vi "_cameras_right_hand_camera_image(Jed)Subscriber_Server.vi"() -> ()   [LabVIEW 2012]
uses:
  <userlib>/rosforlv/ROS/Code/SubVIs/_ROSControl.ctl
  <userlib>/rosforlv/ROS/Code/SubVIs/_ROSDirection.ctl
  <userlib>/rosforlv/ROS/Code/Console/Servers/ServerSubs/ROSLog.ctl
  <userlib>/rosforlv/ROS/Code/Console/Servers/ServerSubs/MyState.ctl
  <userlib>/rosforlv/ROS/Code/Console/Servers/ServerSubs/requestTopic.ctl
panel:
  out "Log of port":string
  out "Queue log":string
  out "Last Reply":string
  out "Registered topics":T1[](array[typedef])
  out "Registering":bool
  out "MyState":T3
  out "(Un)Reg Text":string
  out "Setup":string
  out "Cmd Log":T4[](array[typedef])
  out "Connections Error log":string
  out "Connections":T5(array[cluster])
  out "Error log":string
  in  "stop":bool
  in  "ROS":T1={"topic port"=1236, "Node"="/labview", "topic"="/robot/head/command_head_nod", "type"="std_msgs/Bool", "node port"=7000, "error "={"status"=FALSE, "code"=0, "source"=""}, "Direction"=enum."Publisher", "APIs"=[], "Update (ms)"=1, "write queue"=1}
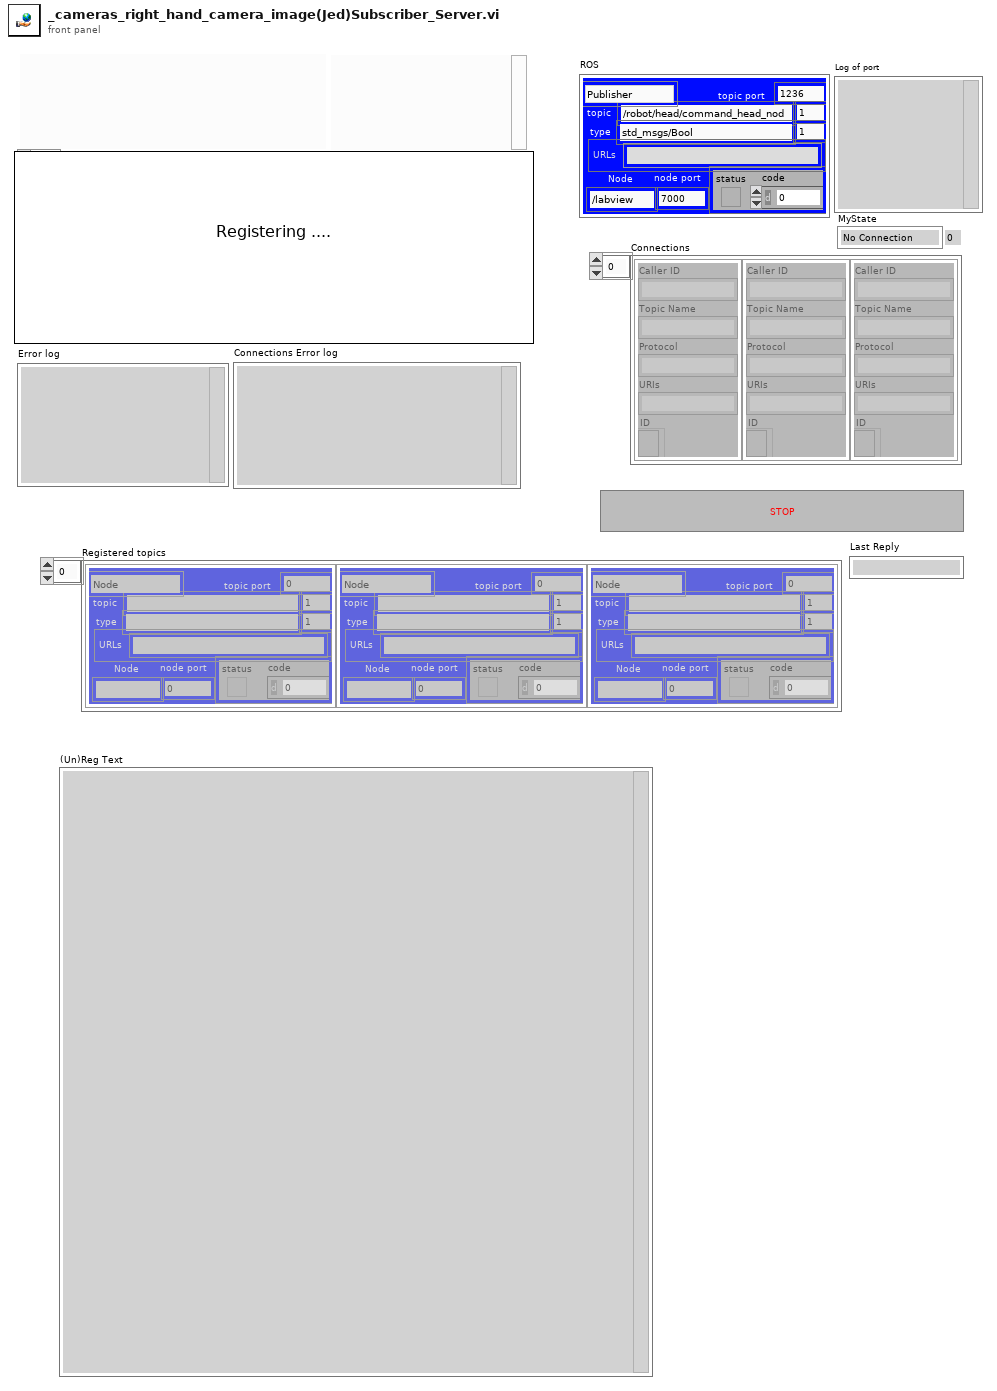
[diagram p1: front panel]
types:
  T1 = typedef "_ROSControl.ctl" = cluster{"topic port":u16, "Node":string, "topic":string, "type":string, "node port":u32, "error ":errorcluster, "Direction":T2, "APIs":string[], "Update (ms)":u16, "write queue":u16}
  T2 = typedef "_ROSDirection.ctl" = enum16{"Node", "Publisher", "Subscriber", "Service Client"}
  T3 = typedef "MyState.ctl" = enum16{"No Connection", "Registered", "Connected", "Close"}
  T4 = typedef "ROSLog.ctl" = cluster{"Sent":string, "Reply":string, "MethodName":string, "success":bool, "Dir1":string, "Dir2":string, "Time Stamp":string}
  T5 = cluster{"Caller ID":string, "Topic Name":string, "Protocol":string, "URIs":string, "ID":refnum<k5>}[]
  T6 = typedef "requestTopic.ctl" = cluster{"New Subscriber":cluster{"Caller ID":string, "Topic Name":string, "Protocol":string, "URIs":string, "ID":refnum<k5>}, "ROS of Server":T1, "new port":u16}
  T7 = cluster{"Code":i32, "Status Message":string, "APIs":string[]}
  T8 = cluster{"Caller ID":string, "Topic Name":string, "Protocol":string, "URIs":string, "ID":refnum<k5>}
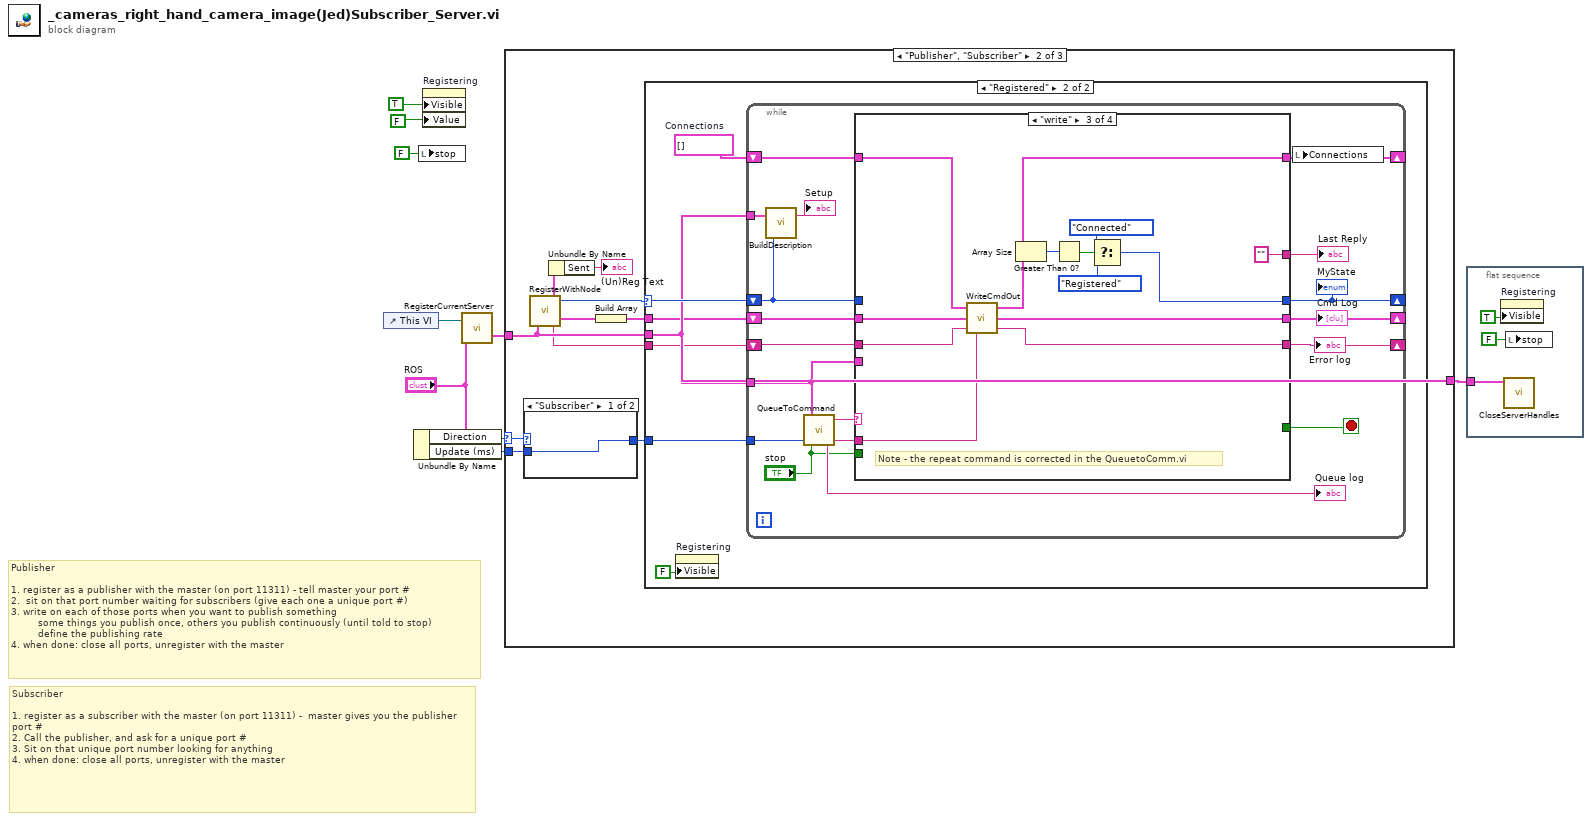
[diagram p0: block diagram]
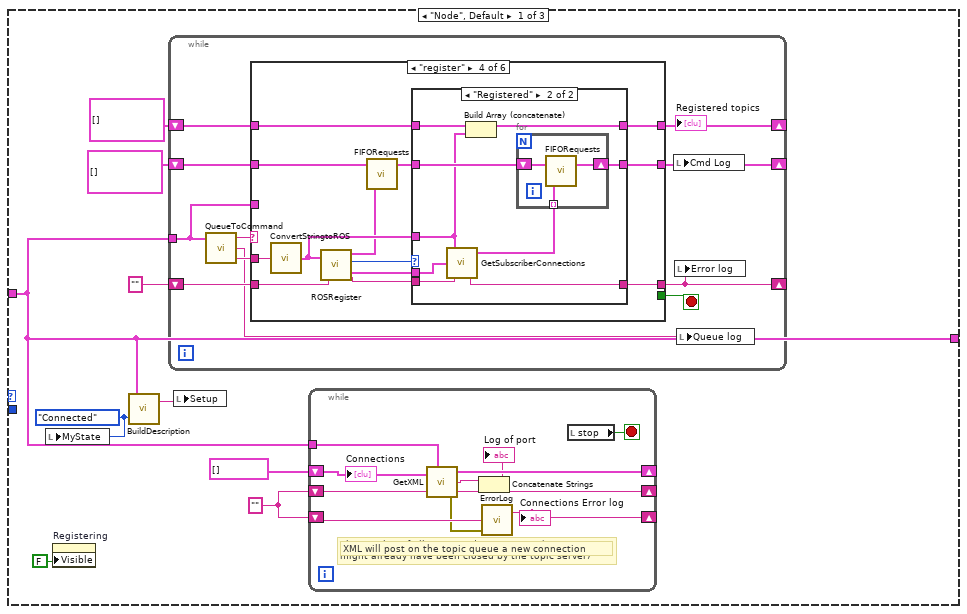
[diagram p2: hidden frame]
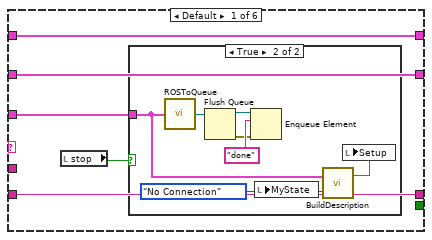
[diagram p3: hidden frame]
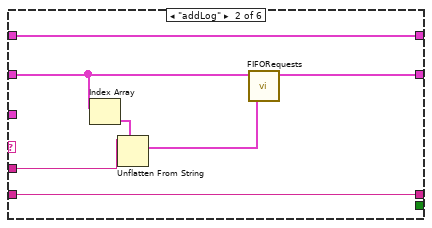
[diagram p5: hidden frame]
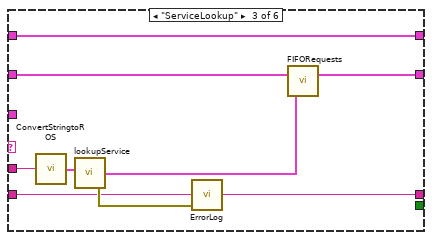
[diagram p6: hidden frame]
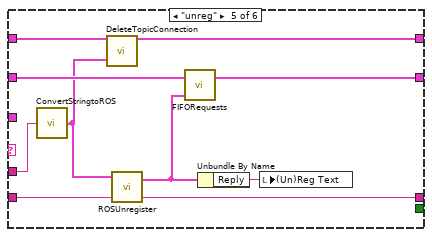
[diagram p8: hidden frame]
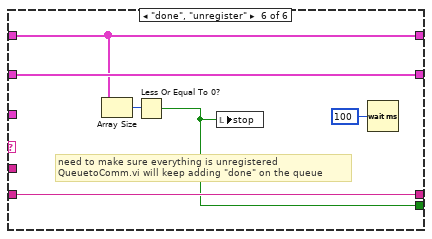
[diagram p9: hidden frame]
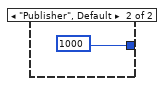
[diagram p10: hidden frame]
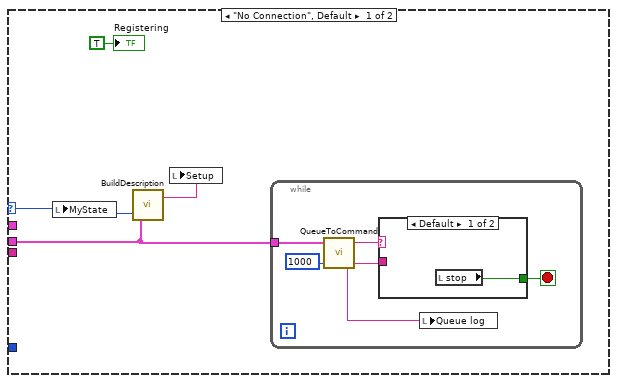
[diagram p11: hidden frame]
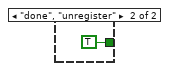
[diagram p12: hidden frame]
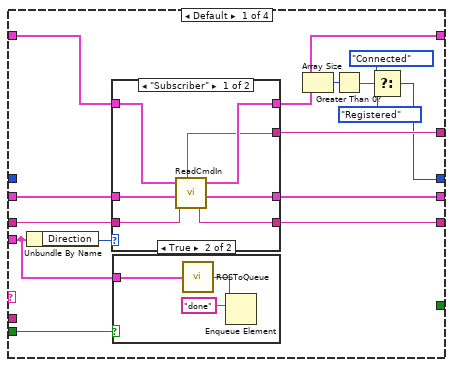
[diagram p13: hidden frame]
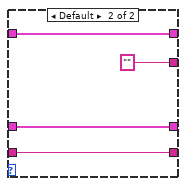
[diagram p14: hidden frame]
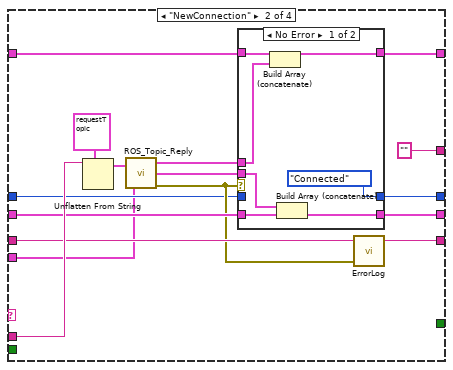
[diagram p16: hidden frame]
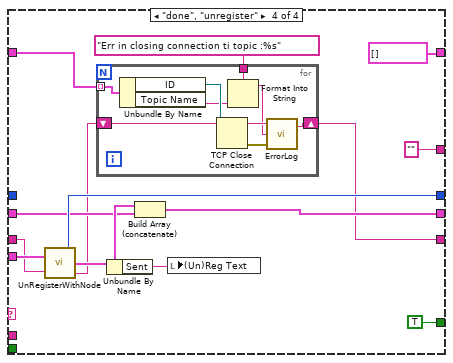
[diagram p18: hidden frame]
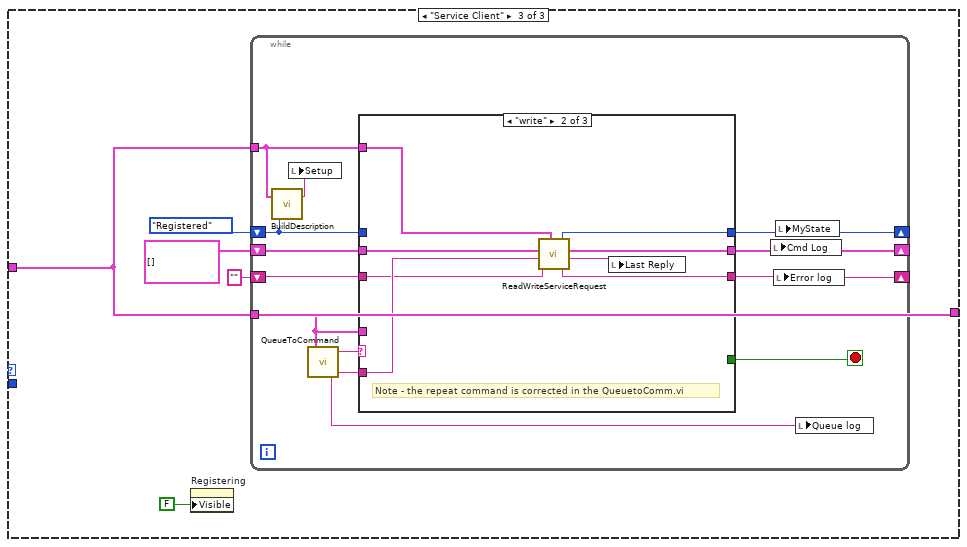
[diagram p19: hidden frame]
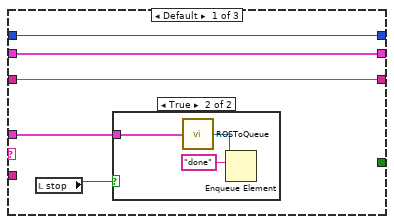
[diagram p20: hidden frame]
diagram:
  # "Subscriber\n\n1. register as a subscriber with the master (on port 11311) -  master gives you the publisher port #\n2. Call the publisher, and ask for a unique port #\n3. Sit on that unique port number looking for anything\n4. when done: close all ports, unregister with the master"
  # "Publisher\n\n1. register as a publisher with the master (on port 11311) - tell master your port #\n2.  sit on that port number waiting for subscribers (give each one a unique port #)\n3. write on each of those ports when you want to publish something\n         some things you publish once, others you publish continuously (until told to stop)\n         define the publishing rate\n4. when done: close all ports, unregister with the master"
  n1 = control-ref of="This VI"() -> (w4:refnum<vi>)
  n2 = Unbundle By Name("ROS") -> ("Direction"=w7:T2, "Update (ms)"=w1:u16)
  n3 = local write "stop"(FALSE ("stop")) -> ()
  n4 = property on="Registering" class="Bool (strict)"("Visible"=TRUE ("Registering"), "Value"=FALSE ("Registering")) -> ()  [unwired: 2 in, 2 out]
  n5 = call <userlib>:"RegisterCurrentServer.vi"("ROS in"="ROS", "This VI"=w4) -> ("ROS out"=w2:T1)  [unwired: 1 in]
  n6 = case shown="\"Publisher\", \"Subscriber\"" w7 {
    selector: w7 -> [_ w117 _]
    tunnel: w2 -> [w12 w120 w254]
    tunnel: [w12 w120 w254] -> w5
    tunnel: w1 -> [_ w112 _]
    frame "Node", Default {
      w11 = "" ("String out")
      w16 = MyState."Connected" ("MyState")
      n7 = local write "MyState"(w16) -> ()
      n8 = property on="Registering" class="Bool (strict)"("Visible"=FALSE ("Registering")) -> ()  [unwired: 2 in, 2 out]
      n9 = call <userlib>:"BuildDescription.vi"("MyState"=w16, "ROS in"=w12) -> ("Setup"=w17:string)  [unwired: 1 in]
      n10 = while {
        shift-right: [w27] -> _
        shift-left: "" ("String out") -> [w28]
        shift-right: [w26] -> _
        shift-left: T4[] [] ("Requests Out") -> [w25]
        shift-right: [w24] -> _
        shift-left: T1[] [] -> [w23]
        tunnel: w12 -> [w19]
        stop <- w29 stop-if-true
        n11 = call <userlib>:"QueueToCommand.vi"("ROS"=w19) -> ("data"=w21:string, "Queue log"=w20:string, "Command"=w22:string)  [unwired: 2 in]
        n12 = case shown="\"register\"" w22 {
          tunnel: [_ _ _ _ _ w97] -> w29
          tunnel: w21 -> [_ w46 w56 w70 w95 _]
          tunnel: w28 -> [w34 w48 w53 w69 w94 w101]
          tunnel: [w34 w48 w52 w58 w93 w101] -> w27
          tunnel: [w33 w42 w49 w68 w90 w100] -> w26
          tunnel: w25 -> [w33 w43 w50 w61 w91 w100]
          tunnel: [w32 w47 w57 w66 w87 w99] -> w24
          tunnel: w23 -> [w32 w47 w57 w67 w88 w99]
          tunnel: w19 -> [w30 _ _ _ _ _]
          frame Default {
            n13 = local read "stop"() -> (w31:bool)
            n14 = case shown="True" w31 {
              tunnel: w30 -> [_ w36]
              frame False {
              }
              frame True {
                w37 = MyState."No Connection" ("MyState")
                n15 = call <userlib>:"ROSToQueue.vi"("ROS"=w36) -> ("queue"=w39:refnum<queue>)  [unwired: 3 in, 1 out]
                n16 = Flush Queue(queue=w39) -> (queue out=w35:refnum<queue>, error out=w40:errorcluster)  [unwired: 1 in, 1 out]
                n17 = Enqueue Element(queue=w35, element="done" ("regular expression"), error in (no error)=w40) -> ()  [unwired: 1 in, 3 out]
                n18 = local write "MyState"(w37) -> ()
                n19 = call <userlib>:"BuildDescription.vi"("MyState"=w37, "ROS in"=w36) -> ("Setup"=w38:string)  [unwired: 1 in]
                n20 = local write "Setup"(w38) -> ()
              }
            }
          }
          frame "addLog" {
            n21 = Index Array(array=w43) -> (element=w45:T4)  [unwired: 1 in]
            n22 = Unflatten From String(type=w45, binary string=w46) -> (value=w44:T4)  [unwired: 3 in, 2 out]
            n23 = call <userlib>:"FIFORequests.vi"("Log"=w44, "Requests in"=w43) -> ("Requests out"=w42:T4[])  [unwired: 1 in]
          }
          frame "ServiceLookup" {
            n24 = call <userlib>:"ConvertStringtoROS.vi"("string in"=w56) -> ("ROS"=w55:T1)
            n25 = call <userlib>:"lookupService.vi"("Service ROS"=w55) -> ("error out"=w54:errorcluster, "Log"=w51:T4)  [unwired: 3 in]
            n26 = call <userlib>:"ErrorLog.vi"("error in"=w54, "String in"=w53) -> ("String out"=w52:string)  [unwired: 1 in, 1 out]
            n27 = call <userlib>:"FIFORequests.vi"("Log"=w51, "Requests in"=w50) -> ("Requests out"=w49:T4[])  [unwired: 1 in]
          }
          frame "register" {
            n28 = call <userlib>:"ConvertStringtoROS.vi"("string in"=w70) -> ("ROS"=w65:T1)
            n29 = call <userlib>:"ROSRegister.vi"("Err In"=w69, "ROS to register"=w65) -> ("Err Out"=w59:string, "Response"=w64:T7, "MyState"=w63:T3, "Log"=w62:T4)
            n30 = call <userlib>:"FIFORequests.vi"("Log"=w62, "Requests in"=w61) -> ("Requests out"=w60:T4[])  [unwired: 1 in]
            n31 = case shown="\"Registered\"" w63 {
              tunnel: w60 -> [w72 w82]
              tunnel: [w72 w81] -> w68
              tunnel: w67 -> [w73 w80]
              tunnel: [w73 w79] -> w66
              tunnel: w65 -> [_ w77]
              tunnel: w64 -> [_ w76]
              tunnel: w59 -> [w71 w75]
              tunnel: [w71 w74] -> w58
              frame Default {
              }
              frame "Registered" {
                n32 = call <userlib>:"GetSubscriberConnections.vi"("Err in"=w75, "Response"=w76, "ROS registered"=w77) -> ("Err out"=w74:string, "Logs out"=w78:T4[])  [unwired: 1 out]
                n33 = Build Array (concatenate)(w80, w77) -> (w79:T1[])
                n34 = for {
                  tunnel: w78 -> [w83] mode=indexing
                  shift-right: [w84] -> w81
                  shift-left: w82 -> [w85]
                  n35 = call <userlib>:"FIFORequests.vi"("Log"=w83, "Requests in"=w85) -> ("Requests out"=w84:T4[])  [unwired: 1 in]
                }
              }
            }
          }
          frame "unreg" {
            n36 = call <userlib>:"ConvertStringtoROS.vi"("string in"=w95) -> ("ROS"=w86:T1)
            n37 = call <userlib>:"DeleteTopicConnection.vi"("ROS"=w86, "Con In"=w88) -> ("Con out"=w87:T1[])
            n38 = call <userlib>:"ROSUnregister.vi"("Err in"=w94, "Server ROS"=w86) -> ("Err out"=w93:string, "Log"=w89:T4)  [unwired: 1 in]
            n39 = call <userlib>:"FIFORequests.vi"("Log"=w89, "Requests in"=w91) -> ("Requests out"=w90:T4[])  [unwired: 1 in]
            n40 = Unbundle By Name(w89) -> ("Reply"=w92:string)
            n41 = local write "(Un)Reg Text"(w92) -> ()
          }
          frame "done", "unregister" {
            # "need to make sure everything is unregistered\nQueuetoComm.vi will keep adding \"done\" on the queue"
            n42 = Array Size(array=w99) -> (size(s)=w98:i32)
            n43 = Less Or Equal To 0?(x=w98) -> (x <= 0?=w97:bool)
            n44 = local write "stop"(w97) -> ()
            n45 = Wait (ms)(milliseconds to wait=u32 100) -> ()  [unwired: 1 out]
          }
        }
        "Registered topics" <- w24
        n46 = local write "Cmd Log"(w26) -> ()
        n47 = local write "Error log"(w27) -> ()
        n48 = local write "Queue log"(w20) -> ()
      }
      n49 = local write "Setup"(w17) -> ()
      n50 = while {
        shift-right: [w111] -> _
        shift-left: T5 [] ("Subscribers") -> [w102]
        tunnel: w12 -> [w109]
        shift-right: [w106] -> _
        shift-left: w11 -> [w110]
        shift-right: [w103] -> _
        shift-left: w11 -> [w105]
        stop <- w107 stop-if-true
        # "This is a log of all requested connections (some\nmight already have been closed by the topic server)"
        # "XML will post on the topic queue a new connection"
        n51 = call <userlib>:"GetXML.vi"("Node ROS"=w109, "Subscribers in"=w102) -> ("error IO"=w108:errorcluster, "reply"=w104:string, "Subscribers Out"=w111:T5)
        n52 = Concatenate Strings(w104, w105) -> (w103:string)
        "Log of port" <- w103
        n53 = call <userlib>:"ErrorLog.vi"("error in"=w108, "String in"=w110) -> ("String out"=w106:string)  [unwired: 1 in, 1 out]
        "Connections Error log" <- w106
        n54 = local read "stop"() -> (w107:bool)
        "Connections" <- w102
      }
    }
    frame "Publisher", "Subscriber" {
      n55 = case shown="\"Subscriber\"" w117 {
        tunnel: [w121 1000 ("timeout in ms (1000)")] -> w116
        tunnel: w112 -> [w121 _]
        frame "Subscriber" {
        }
        frame "Publisher", Default {
        }
      }
      n56 = call <userlib>:"RegisterWithNode.vi"("ROS"=w120) -> ("MyState"=w118:T3, "Log"=w115:T4, "Error"=w113:string)
      n57 = Unbundle By Name(w115) -> ("Sent"=→"(Un)Reg Text":string)
      n58 = Build Array(w115) -> (w114:T4[])
      n59 = case shown="\"Registered\"" w118 {
        selector: w118 -> [w125 w140]
        tunnel: w120 -> [w123 w138]
        tunnel: w116 -> [_ w137]
        tunnel: w114 -> [_ w136]
        tunnel: w113 -> [_ w135]
        frame "No Connection", Default {
          n60 = local write "MyState"(w125) -> ()
          n61 = call <userlib>:"BuildDescription.vi"("MyState"=w125, "ROS in"=w123) -> ("Setup"=w126:string)  [unwired: 1 in]
          n62 = local write "Setup"(w126) -> ()
          n63 = while {
            tunnel: w123 -> [w127]
            stop <- w132 stop-if-true
            n64 = call <userlib>:"QueueToCommand.vi"("timeout"=1000 ("timeout in ms (-1)"), "ROS"=w127) -> ("data"=w131:string, "Queue log"=w128:string, "Command"=w129:string)  [unwired: 1 in]
            n65 = case shown="Default" w129 {
              tunnel: [w133 TRUE] -> w132
              tunnel: w131 -> [_ _]
              frame Default {
                n66 = local read "stop"() -> (w133:bool)
              }
              frame "done", "unregister" {
              }
            }
            n67 = local write "Queue log"(w128) -> ()
          }
          "Registering" <- TRUE ("Registering")
        }
        frame "Registered" {
          w141 = T5 []  # Connections
          n68 = property on="Registering" class="Bool (strict)"("Visible"=FALSE ("Registering")) -> ()  [unwired: 2 in, 2 out]
          n69 = while {
            shift-right: [w158] -> _
            shift-left: w135 -> [w159]
            shift-right: [w155] -> _
            shift-left: w136 -> [w156]
            shift-right: [w153] -> _
            shift-left: w140 -> [w144]
            tunnel: w138 -> [w152]
            tunnel: w138 -> [w143]
            shift-right: [w146] -> _
            shift-left: w141 -> [w151]
            tunnel: w137 -> [w145]
            stop <- w150 stop-if-true
            n70 = call <userlib>:"BuildDescription.vi"("MyState"=w144, "ROS in"=w152) -> ("Setup"=→"Setup":string)  [unwired: 1 in]
            n71 = call <userlib>:"QueueToCommand.vi"("timeout"=w145, "Stop Btn Pressed?"="stop", "ROS"=w143) -> ("data"=w157:string, "Queue log"=→"Queue log":string, "Command"=w148:string)
            n72 = case shown="\"write\"" w148 {
              tunnel: [w172 w194 w227 w233] -> w158
              tunnel: w159 -> [w171 w195 w226 w230]
              tunnel: [w163 w192 w217 w241] -> w153
              tunnel: w157 -> [_ w200 w223 _]
              tunnel: w156 -> [w170 w198 w225 w236]
              tunnel: [w173 w197 w224 w235] -> w155
              tunnel: w151 -> [w169 w204 w221 w234]
              tunnel: [w164 w203 w215 T5 [] ("Connections Out")] -> w146
              tunnel: [_ _ _ TRUE] -> w150
              tunnel: [w174 "" ("String out") "" ("String out") "" ("String out")] -> w149
              tunnel: w144 -> [_ w191 _ _]
              tunnel: w143 -> [w161 w189 _ w231]
              tunnel: "stop" -> [w160 _ _ _]
              frame Default {
                n73 = Unbundle By Name(w161) -> ("Direction"=w162:T2)
                n74 = case shown="\"Subscriber\"" w162 {
                  tunnel: [w176 "" ("String out")] -> w174
                  tunnel: [w181 w182] -> w164
                  tunnel: [w180 w184] -> w173
                  tunnel: [w179 w183] -> w172
                  tunnel: w171 -> [w178 w183]
                  tunnel: w170 -> [w177 w184]
                  tunnel: w169 -> [w175 w182]
                  frame "Subscriber" {
                    n75 = call <userlib>:"ReadCmdIn.vi"("Connections"=w175, "Log in"=w177, "Err in"=w178) -> ("data"=w176:string, "Connections out"=w181:T5, "Log out"=w180:T4[], "Err out"=w179:string)  [unwired: 1 in]
                  }
                  frame Default {
                  }
                }
                n76 = case shown="True" w160 {
                  tunnel: w161 -> [_ w186]
                  frame False {
                  }
                  frame True {
                    n77 = call <userlib>:"ROSToQueue.vi"("ROS"=w186) -> ("queue"=w187:refnum<queue>)  [unwired: 3 in, 1 out]
                    n78 = Enqueue Element(queue=w187, element="done") -> ()  [unwired: 2 in, 3 out]
                  }
                }
                n79 = Array Size(array=w164) -> (size(s)=w168:i32)
                n80 = Greater Than 0?(x=w168) -> (x > 0?=w165:bool)
                n81 = Select(t=MyState."Connected" ("f"), s=w165, f=MyState."Registered") -> (s? t:f=w163:T3)
              }
              frame "NewConnection" {
                n82 = Unflatten From String(type=T6 {"New Subscriber"={"Caller ID"="", "Topic Name"="", "Protocol"="", "URIs"="", "ID"=refnum}, "ROS of Server"={"topic port"=0, "Node"="", "topic"="", "type"="", "node port"=0, "error "={"status"=FALSE, "code"=0, "source"=""}, "Direction"=enum."Node", "APIs"=[], "Update (ms)"=0, "write queue"=0}, "new port"=0} ("data"), binary string=w200) -> (value=w196:T6)  [unwired: 3 in, 2 out]
                n83 = call <userlib>:"ROS_Topic_Reply.vi"("data"=w196, "My ROS"=w189) -> ("Subscriber out"=w201:T8, "Log"=w199:T4, "error IO"=w193:errorcluster)
                n84 = case shown="No Error" w193 {
                  tunnel: w204 -> [w211 w214]
                  tunnel: [w210 w214] -> w203
                  tunnel: w201 -> [w209 _]
                  tunnel: w199 -> [w208 _]
                  tunnel: w198 -> [w207 w213]
                  tunnel: [w206 w213] -> w197
                  tunnel: [MyState."Connected" ("MyState") w212] -> w192
                  tunnel: w191 -> [_ w212]
                  frame No Error {
                    n85 = Build Array (concatenate)(w211, w209) -> (w210:T5)
                    n86 = Build Array (concatenate)(w208, w207) -> (w206:T4[])
                  }
                  frame Error {
                  }
                }
                n87 = call <userlib>:"ErrorLog.vi"("error in"=w193, "Error String"=w195) -> ("String out"=w194:string)  [unwired: 1 in, 1 out]
              }
              frame "write" {
                # "Note - the repeat command is corrected in the QueuetoComm.vi"
                n88 = call <userlib>:"WriteCmdOut.vi"("Connections In"=w221, "Log in"=w225, "Err in"=w226, "data"=w223) -> ("Connections Out"=w215:T5, "Log out"=w224:T4[], "Err out"=w227:string)  [unwired: 1 in]
                n89 = Array Size(array=w215) -> (size(s)=w216:i32)
                n90 = Greater Than 0?(x=w216) -> (x > 0?=w220:bool)
                n91 = Select(t=MyState."Connected" ("f"), s=w220, f=MyState."Registered") -> (s? t:f=w217:T3)
              }
              frame "done", "unregister" {
                n92 = call <userlib>:"UnRegisterWithNode.vi"("ROS"=w231, "Err in"=w230) -> ("MyState"=w241:T3, "Log"=w237:T4, "Err out"=w229:string)
                n93 = for {
                  tunnel: w234 -> [w249] mode=indexing
                  shift-right: [w247] -> w233
                  shift-left: w229 -> [w246]
                  tunnel: "Err in closing connection ti topic :%s" ("String in") -> [w244]
                  n94 = Unbundle By Name(w249) -> ("ID"=w248:refnum<k5>, "Topic Name"=w243:string)
                  n95 = TCP Close Connection(connection ID=w248) -> (error out=w245:errorcluster)  [unwired: 2 in, 1 out]
                  n96 = Format Into String(format string=w244, w243) -> (resulting string=w242:string)  [unwired: 2 in, 1 out]
                  n97 = call <userlib>:"ErrorLog.vi"("error in"=w245, "String in"=w242, "Error String"=w246) -> ("String out"=w247:string)  [unwired: 1 out]
                }
                n98 = Unbundle By Name(w237) -> ("Sent"=w240:string)
                n99 = Build Array (concatenate)(w237, w236) -> (w235:T4[])
                n100 = local write "(Un)Reg Text"(w240) -> ()
              }
            }
            "Error log" <- w158
            "Cmd Log" <- w155
            "MyState" <- w153
            "Last Reply" <- w149
            n101 = local write "Connections"(w146) -> ()
          }
        }
      }
    }
    frame "Service Client" {
      n102 = property on="Registering" class="Bool (strict)"("Visible"=FALSE ("Registering")) -> ()  [unwired: 2 in, 2 out]
      n103 = while {
        shift-right: [w260] -> _
        shift-left: "" ("String out") -> [w267]
        shift-right: [w259] -> _
        shift-left: T4[] [] ("Log") -> [w265]
        shift-right: [w261] -> _
        shift-left: MyState."Registered" ("MyState") -> [w264]
        tunnel: w254 -> [w256]
        tunnel: w254 -> [w255]
        stop <- w263 stop-if-true
        n104 = call <userlib>:"BuildDescription.vi"("MyState"=w264, "ROS in"=w256) -> ("Setup"=w257:string)  [unwired: 1 in]
        n105 = local write "Setup"(w257) -> ()
        n106 = call <userlib>:"QueueToCommand.vi"("ROS"=w255) -> ("data"=w266:string, "Queue log"=w258:string, "Command"=w262:string)  [unwired: 2 in]
        n107 = case shown="\"write\"" w262 {
          tunnel: [w269 w277 w286] -> w260
          tunnel: w267 -> [w269 w278 w286]
          tunnel: [w271 w281 MyState."No Connection" ("MyState")] -> w261
          tunnel: w266 -> [_ w279 _]
          tunnel: w265 -> [w270 w283 w287]
          tunnel: [w270 w282 w287] -> w259
          tunnel: w264 -> [w271 _ _]
          tunnel: [_ _ TRUE] -> w263
          tunnel: w256 -> [_ w280 _]
          tunnel: w255 -> [w268 _ _]
          frame Default {
            n108 = local read "stop"() -> (w272:bool)
            n109 = case shown="True" w272 {
              tunnel: w268 -> [_ w273]
              frame False {
              }
              frame True {
                n110 = call <userlib>:"ROSToQueue.vi"("ROS"=w273) -> ("queue"=w274:refnum<queue>)  [unwired: 3 in, 1 out]
                n111 = Enqueue Element(queue=w274, element="done") -> ()  [unwired: 2 in, 3 out]
              }
            }
          }
          frame "write" {
            # "Note - the repeat command is corrected in the QueuetoComm.vi"
            n112 = call <userlib>:"ReadWriteServiceRequest.vi"("Service ROS"=w280, "Error in"=w278, "data"=w279, "Log in"=w283) -> ("Error out"=w277:string, "String Read"=w276:string, "Log"=w282:T4[], "MyState"=w281:T3)  [unwired: 1 in]
            n113 = local write "Last Reply"(w276) -> ()
          }
          frame "done", "unregister" {
            # "stop all repeating connections"
          }
        }
        n114 = local write "Cmd Log"(w259) -> ()
        n115 = local write "Error log"(w260) -> ()
        n116 = local write "MyState"(w261) -> ()
        n117 = local write "Queue log"(w258) -> ()
      }
    }
  }
  n118 = flat-sequence {
    tunnel: w5 -> [w288]
    frame #0 {
      n119 = property on="Registering" class="Bool (strict)"("Visible"=TRUE ("Registering")) -> ()  [unwired: 2 in, 2 out]
      n120 = call <userlib>:"CloseServerHandles.vi"("ROS"=w288) -> ()
      n121 = local write "stop"(FALSE ("stop")) -> ()
    }
  }
